vi "Add Control Caption.vi"(8 "error in (no error)":errorcluster, 11 "Combo Box in":refnum<class "Combo Box.lvclass">) -> (0 "error out":errorcluster, 3 "Combo Box out":refnum<class "Combo Box.lvclass">)   [LabVIEW 2017, in "Localization.lvlib" / "Combo Box.lvclass"]
doc: "VI for override that is supposed to do go throgh and create the Caption for the specific VI. Then the caption is set as visible and the label is hidden.\n\nChoose Movement Consulting, LLC"
uses:
  Combo Box.lvclass
  C:/Apps/CMC/OpenSource/Localization/Control Info/Control Info.lvclass
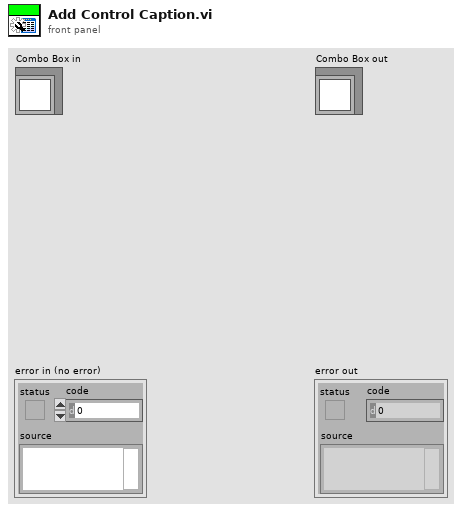
[diagram p1: front panel]
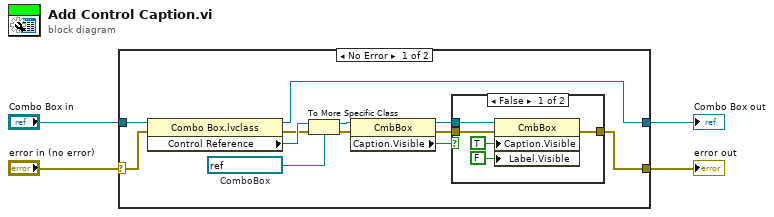
[diagram p0: block diagram]
diagram:
  n1 = case shown="No Error" "error in (no error)" {
    selector: "error in (no error)" -> [w11 w24]
    tunnel: "Combo Box in" -> [w10 w23]
    tunnel: [w7 w23] -> w1
    tunnel: [w5 w24] -> w2
    frame No Error {
      w12 = refnum<vi> refnum  # ComboBox
      n2 = property class="Combo Box.lvclass"(reference=w10, error in=w11) -> (reference out=w7:refnum<class "Combo Box.lvclass">, error out=w15:errorcluster, "Control Reference"=w16:refnum<vi>)
      n3 = To More Specific Class(target class=w12, reference=w16, error in=w15) -> (specific class reference=w13:refnum<vi>, error out=w14:errorcluster)
      n4 = property class="CmbBox"(reference=w13, error in=w14) -> (reference out=w6:refnum<vi>, error out=w8:errorcluster, "Caption.Visible"=w9:bool)
      n5 = case shown="False" w9 {
        tunnel: w8 -> [w20 w22]
        tunnel: w6 -> [w21 _]
        tunnel: [w17 w22] -> w5
        frame False {
          n6 = property class="CmbBox"(reference=w21, error in=w20, "Caption.Visible"=TRUE, "Label.Visible"=FALSE) -> (error out=w17:errorcluster)  [unwired: 1 out]
        }
        frame True {
        }
      }
    }
    frame Error {
    }
  }
  "error out" <- w2
  "Combo Box out" <- w1
